vi "Read listenner.vi"(8 "error in (no error)":errorcluster, 11 "Server in":refnum<class "TCP-Server.lvclass">) -> (0 "error out":errorcluster, 2 "listenner ID":refnum<k5>, 3 "Server out":refnum<class "TCP-Server.lvclass">)   [LabVIEW 2018, in "TCP-Server.lvclass"]
uses:
  TCP-Server.lvclass
  TCP-Server.lvclass/TCP-Server.ctl
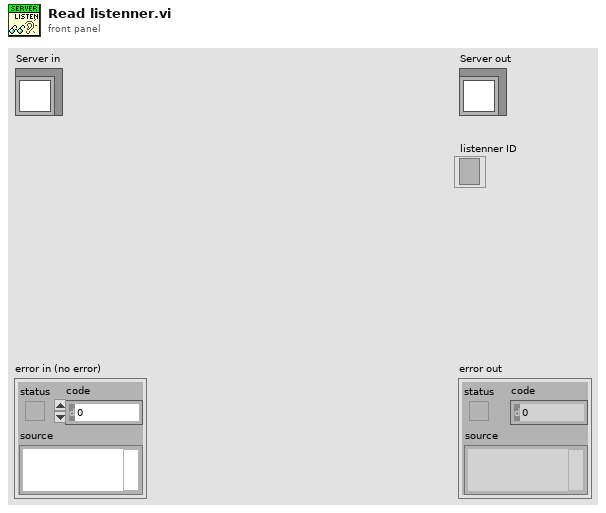
[diagram p1: front panel]
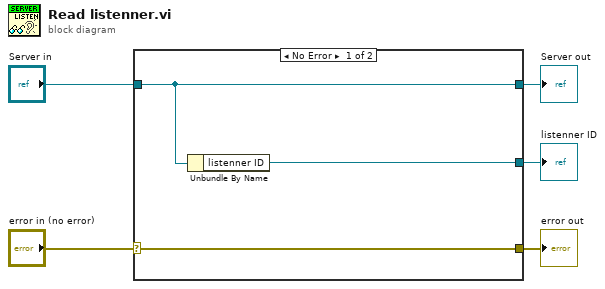
[diagram p0: block diagram]
diagram:
  n1 = case shown="No Error" "error in (no error)" {
    selector: "error in (no error)" -> [w8 w9]
    tunnel: [w8 w9] -> w4
    tunnel: [w6 w10] -> w2
    tunnel: "Server in" -> [w6 w10]
    tunnel: [w7 _] -> w1
    frame No Error {
      n2 = Unbundle By Name(w6) -> ("listenner ID"=w7:refnum<k5>)
    }
    frame Error {
    }
  }
  "error out" <- w4
  "Server out" <- w2
  "listenner ID" <- w1
